vi "CameraGetInfo.vi"(8 "error in (no error)":errorcluster, 11 "CameraBase in":refnum<class "CameraBase.lvclass">) -> (0 "error out":errorcluster, 1 "serial":u64, 2 "name":string, 3 "CameraBase out":refnum<class "CameraBase.lvclass">, 5 "location":string)   [LabVIEW 2012, in "CameraBase.lvclass"]
uses:
  <userlib>/BIAS2/classes/CameraBase/CameraBase.lvclass
  <userlib>/BIAS2/classes/CameraBase/CameraBase.lvclass/CameraBase.ctl
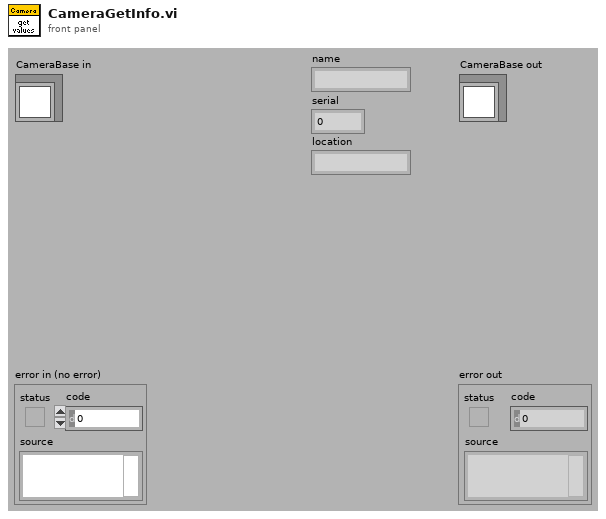
[diagram p1: front panel]
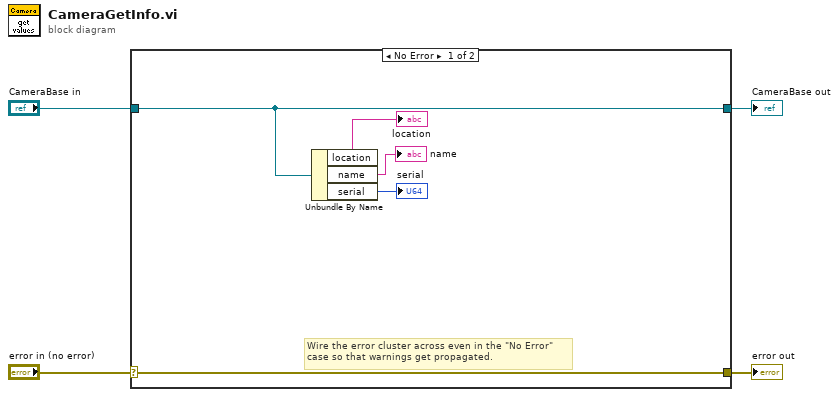
[diagram p0: block diagram]
diagram:
  n1 = case shown="No Error" "error in (no error)" {
    selector: "error in (no error)" -> [w9 w11]
    tunnel: [w9 w11] -> w3
    tunnel: [w8 w10] -> w1
    tunnel: "CameraBase in" -> [w8 w10]
    frame No Error {
      # "Wire the error cluster across even in the \"No Error\"\ncase so that warnings get propagated."
      n2 = Unbundle By Name(w8) -> ("location"=→"location":string, "name"=→"name":string, "serial"=→"serial":u64)
    }
    frame Error {
    }
  }
  "error out" <- w3
  "CameraBase out" <- w1
